vi "Default Instrument Setup.vi"(8 "error in (no error)":errorcluster, 11 "VISA resource name":refnum<visa-resource-name>) -> (0 "error out":errorcluster, 3 "VISA resource name out":refnum<visa-resource-name>)   [LabVIEW 2010, in "Agilent 3458.lvlib"]
doc: "Sets the instrument to a state that allows to start taking measurements. First the instrument is presetted, then the memory input and output formats is set to single real (which requires only 4 bytes per measurements). The input buffer is turned off so that every command is processed without being interrupted, the status byte register is cleared, delay between samples is set to auto, memory is set to first in first out mode, the trigger buffer is turned on to prevent the trigger too fast error, the number of integration cycles is set to 10 and finally the number of digits displayed is set to 8.5."
uses:
  <instrlib>/Agilent 3458/Agilent 3458.lvlib
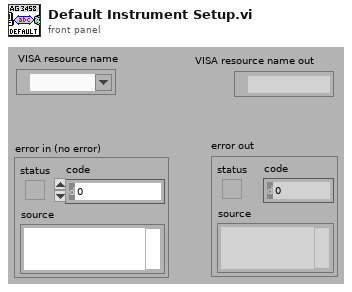
[diagram p1: front panel]
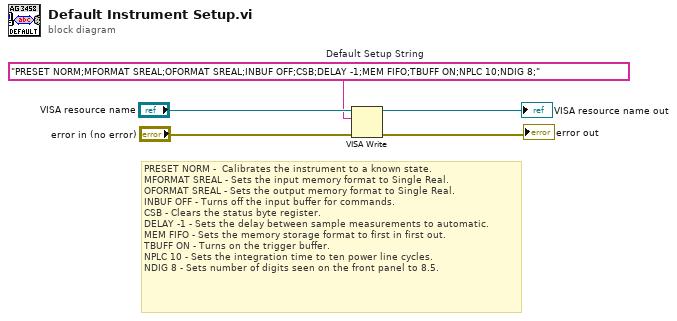
[diagram p0: block diagram]
diagram:
  w3 = "PRESET NORM;MFORMAT SREAL;OFORMAT SREAL;INBUF OFF;CSB;DELAY -1;MEM FIFO;TBUFF ON;NPLC 10;NDIG 8;"  # Default Setup String
  # "PRESET NORM -  Calibrates the instrument to a known state.\nMFORMAT SREAL - Sets the input memory format to Single Real.\nOFORMAT SREAL - Sets the output memory format to Single Real.\nINBUF OFF - Turns off the input buffer for commands.\nCSB - Clears the status byte register.\nDELAY -1 - Sets the delay between sample measurements to automatic.\nMEM FIFO - Sets the memory storage format to first in first out.\nTBUFF ON - Turns on the trigger buffer.\nNPLC 10 - Sets the integration time to ten power line cycles.\nNDIG 8 - Sets number of digits seen on the front panel to 8.5."
  n1 = VISA Write(VISA resource name="VISA resource name", write buffer=w3, error in (no error)="error in (no error)") -> (VISA resource name out=→"VISA resource name out":refnum<visa-resource-name>, error out=→"error out":errorcluster)  [unwired: 1 out]
